vi "ManualMotorControl.vi"() -> ()   [LabVIEW 2021]
uses:
  Controls/Status Lights.ctl
  <vilib>/event_ctls.llb/eventsource.ctl
  <vilib>/event_ctls.llb/lveventtype.ctl
  <vilib>/event_ctls.llb/eventvkey.ctl
  Controls/ManualConttrolCluster.ctl
  Controls/State Machine Data.ctl
  Controls/DAQ Refnums.ctl
  <vilib>/Utility/error.llb/Error Cluster From Error Code.vi
  <vilib>/ErrorRing/Error Ring.xnode
panel:
  in  "Manual Control Cluster":T1 {"Speed" scale=0.0..5.0}
  out "Extend":bool
  out "Stop Button":bool
  out "Retract":bool
  out "Char":i16
  out "VKey":T2
  out "Type":T3=enum."Value Change"
  out "Source":T4 items=["LabVIEW UI"=0, "ActiveX"=1, "User Event"=25]
  out "Mods":cluster{"Num Pad":bool, "Menu Key":bool}
  out "PlatMods":T5
  out "Time":u32
  out "ScanCode":i16
  in  "Simulated Pressure":dbl
  out "Speed":dbl
  out "Actuator Status":T6
  out "Pressure MPa":dbl
  in  "Target Pressure MPa":dbl
  out "Control State":string
  in  "Simulate":bool
  in  "Exit Button":bool
  out "error out":errorcluster
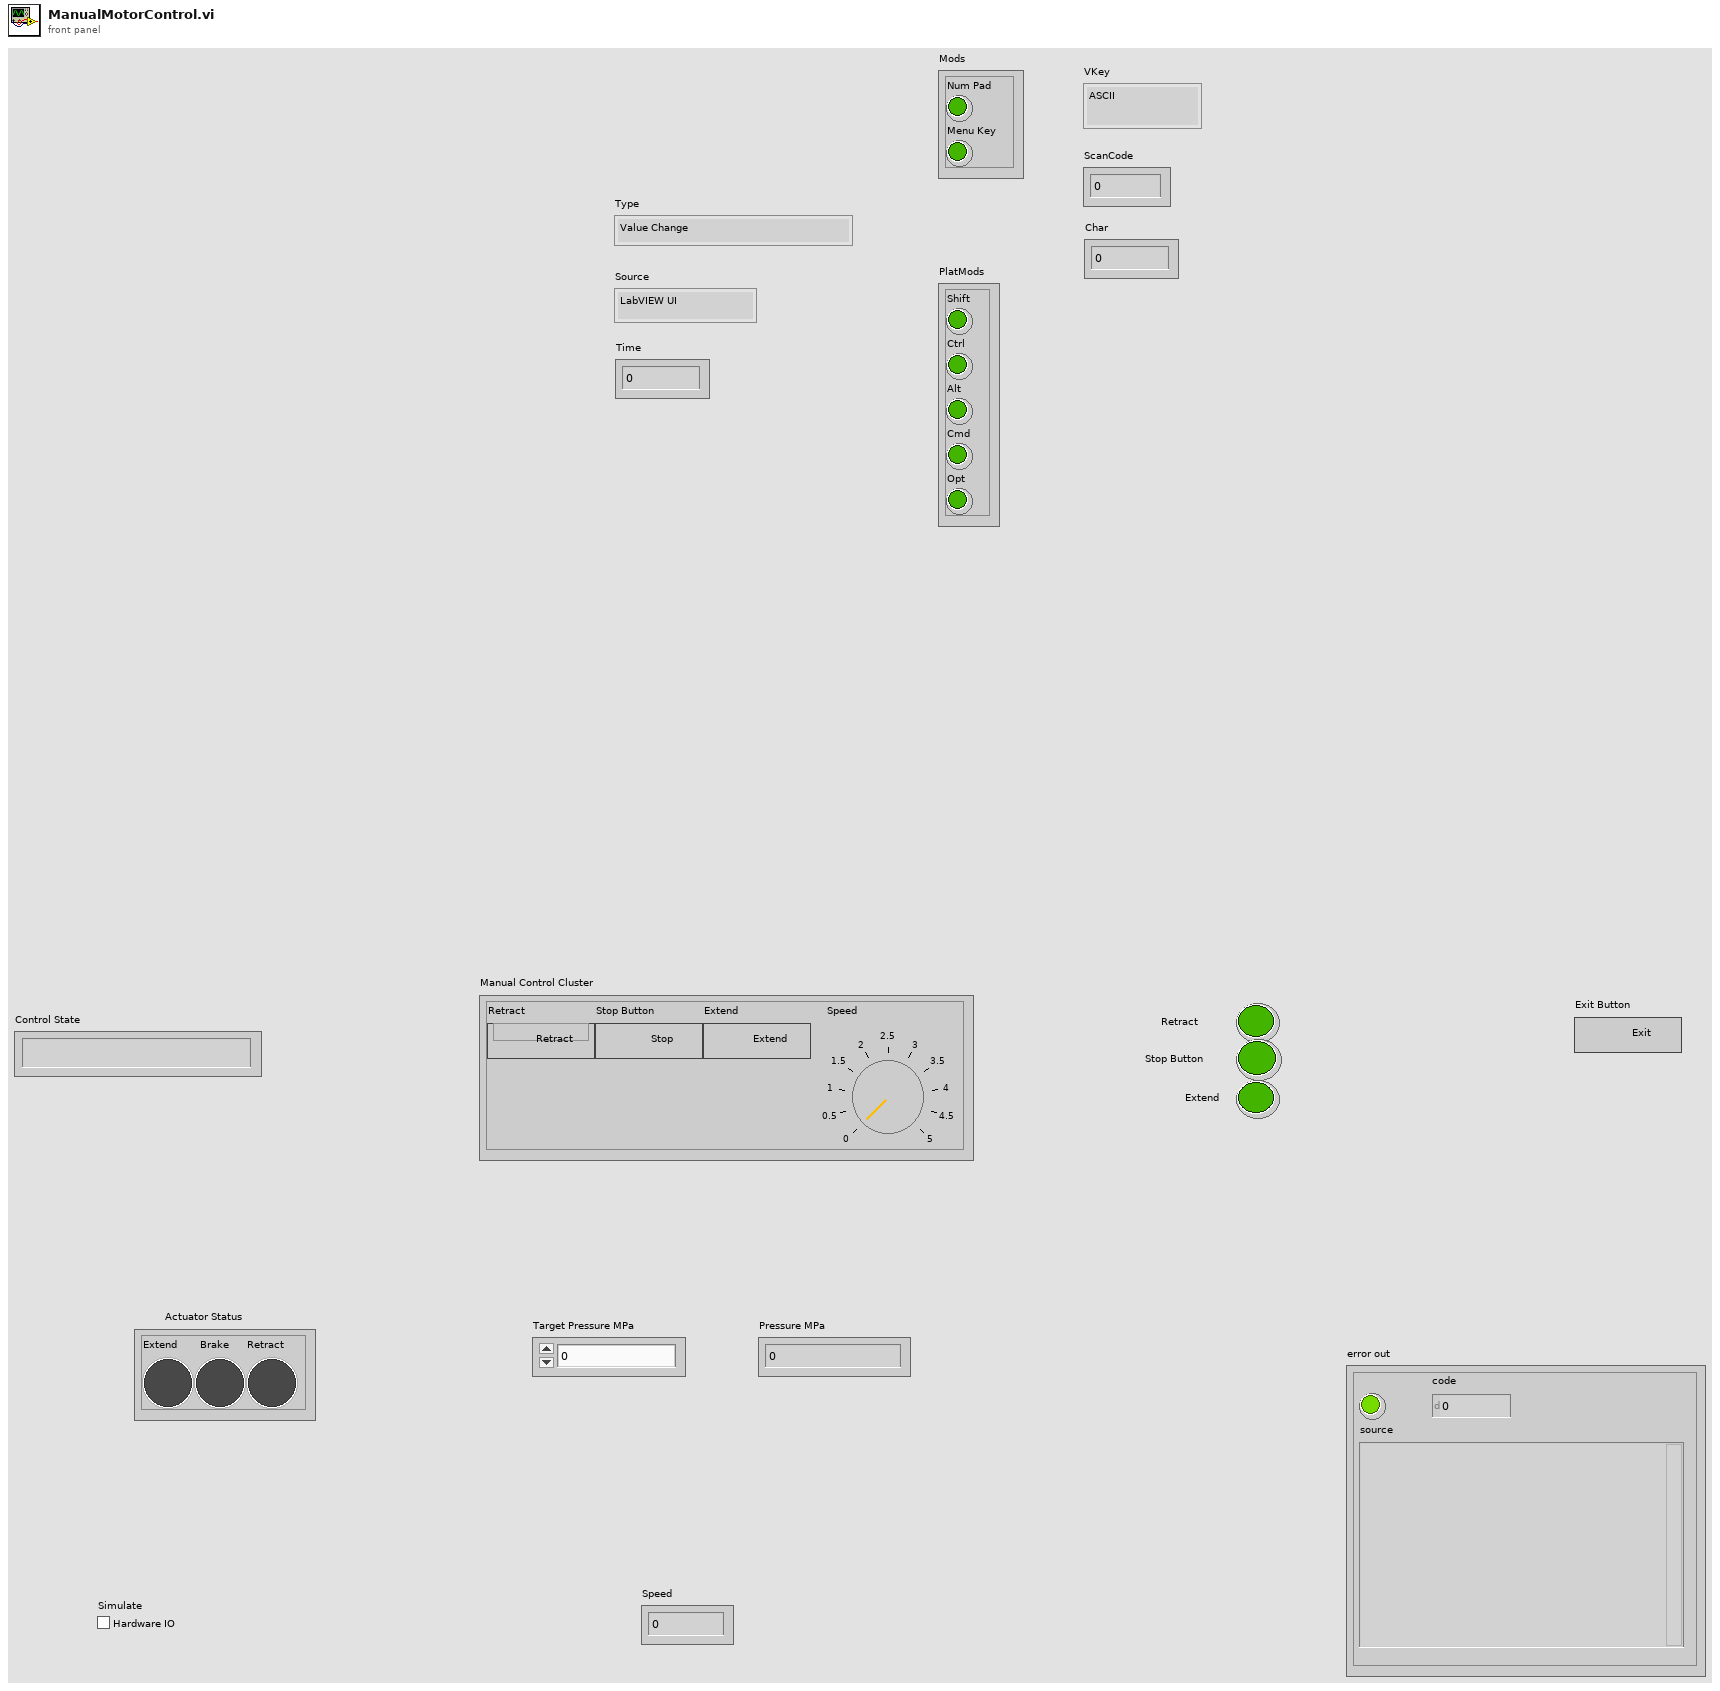
[diagram p1: front panel]
types:
  T1 = typedef "ManualConttrolCluster.ctl" = cluster{"Retract":bool, "Stop Button":bool, "Extend":bool, "Speed":dbl}
  T2 = typedef "eventvkey.ctl" = enum16{"ASCII", "Enter", "Return", "Shift", "Ctrl", "Alt", "Cmd", "Opt", "Caps", "NumLock", "Clear", "Break", "Up", "Down", "Left", "Right", "Insert", "Delete", "Home", "End", "PageUp", "PageDown", "Escape", "Help", "Pause", "ScrollLock", "F1", "F2", "F3", "F4", "F5", "F6", "F7", "F8", "F9", "F10", "F11", "F12", "F13", "F14", "F15", "F16", "F17", "F18", "F19", "F20", "F21", "F22", "F23", "F24", "Play", "VolumeUp", "VolumeDown", "Mute", "Two Byte Char"}
  T3 = typedef "lveventtype.ctl" = enum32{"Null", "Timeout", "Annotation Menu Selection", "Annotation Menu Selection?", "App Instance Close", "App Instance Close?", "Autoscale Range Change", "Bookmark Info Change", "Cell Edit", "Cell Edit?", "Cursor Grab", "Cursor Grab?", "Cursor Menu Selection", "Cursor Menu Selection?", "Cursor Move", "Cursor Release", "Data Change", "Direction Change", "Display State Change", "Drag Ended", "Drag Enter", "Drag Leave", "Drag Over", "Drag Source Update", "Drag Starting", "Drag Starting?", "Drop", "Exec State Change", "Key Down", "Key Down?", "Key Repeat", "Key Repeat?", "Key Up", "Listbox Double Click", "Menu Activation?", "Menu Selection (App)", "Menu Selection? (App)", "Menu Selection (User)", "Mouse Down", "Mouse Down?", "Mouse Enter", "Mouse Leave", "Mouse Move", "Mouse Up", "Mouse Wheel", "NI Security User Change (App)", "Pane Size", "Panel Close", "Panel Close?", "Panel Resize", "Plot Attribute Change", "Scale Range Change", "Shortcut Menu Activation?", "Shortcut Menu Selection (App)", "Shortcut Menu Selection? (App)", "Shortcut Menu Selection (User)", "Tree Double Click", "Tree Drag", "Tree Drag?", "Tree Drop", "Tree Drop?", "Tree Item Close", "Tree Item Close?", "Tree Item Open", "Tree Item Open?", "User Event", "Value Change"}
  T4 = typedef "eventsource.ctl" = u32
  T5 = cluster{"Shift":bool, "Ctrl":bool, "Alt":bool, "Cmd":bool, "Opt":bool}
  T6 = typedef "Status Lights.ctl" = cluster{"Extend":bool, "Brake":bool, "Retract":bool}
  T7 = cluster{"Start Button":refnum<vi>, "Pause Button":refnum<vi>, "Stop Button":refnum<vi>}
  T8 = typedef "State Machine Data.ctl" = cluster{"Control State":string, "Status Message":string, "Speed":dbl, "Pressure":dbl, "Target Pressure":dbl, "Apply Brake Ref":refnum<vi>, "Release Brake Ref":refnum<vi>, "Extend Ref":refnum<vi>, "Retract Ref":refnum<vi>, "Pressure Ref":refnum<vi>, "Data Display Ref":refnum<vi>, "Exit Button Ref":refnum<vi>, "Bool":bool, "Status":T6}
  T9 = typedef "DAQ Refnums.ctl" = cluster{"Direction Ref":refnum<k21>, "Brake Ref":refnum<k21>, "Speed Ref":refnum<k21>, "Pressure Ref":refnum<k21>}
  T10 = typedef "UI Data.ctl" = cluster{"Sampling State":string, "Status Message":string, "Speed":dbl, "Pressure":dbl, "Target Pressure":dbl, "Apply Brake Ref":refnum<vi>, "Release Brake Ref":refnum<vi>, "Extend Ref":refnum<vi>, "Retract Ref":refnum<vi>, "Pressure Ref":refnum<vi>, "Data Display Ref":refnum<vi>, "Exit Button Ref":refnum<vi>, "Speed Pressure Select":bool, "Status":T6}
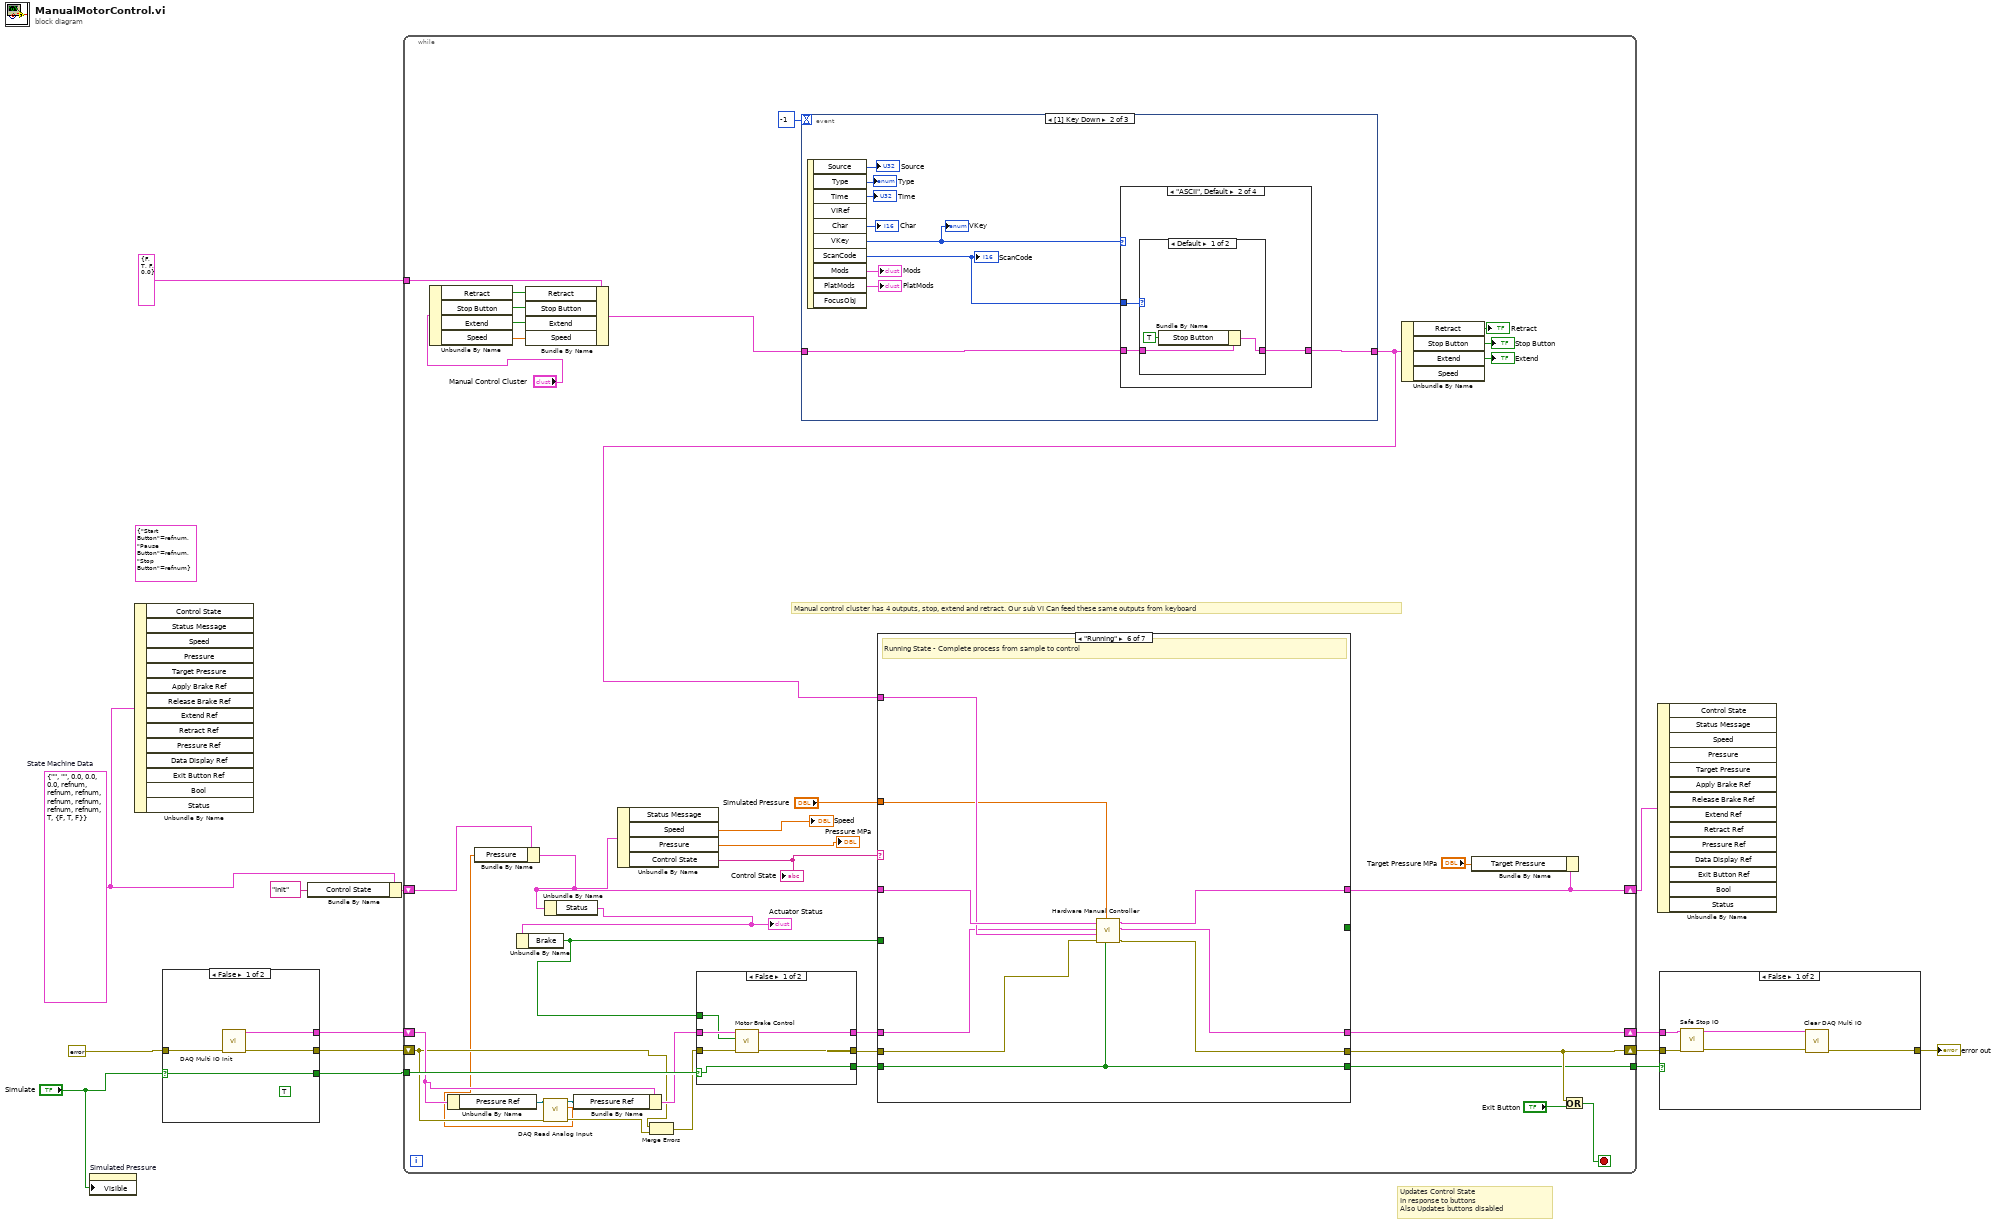
[diagram p0: block diagram]
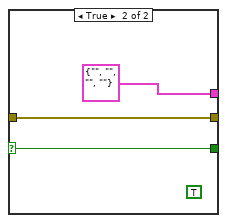
[diagram p3: hidden frame]
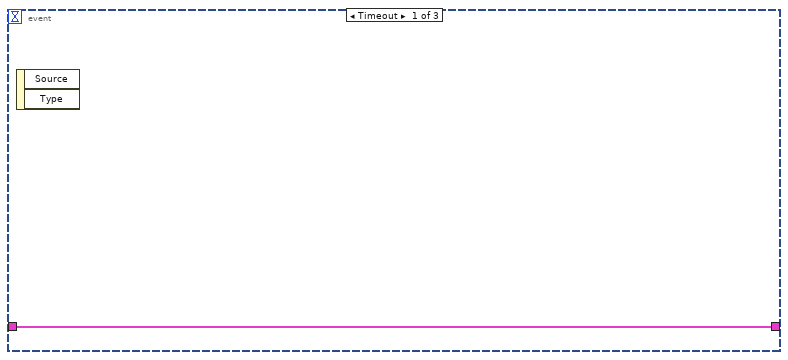
[diagram p4: hidden frame]
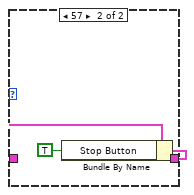
[diagram p6: hidden frame]
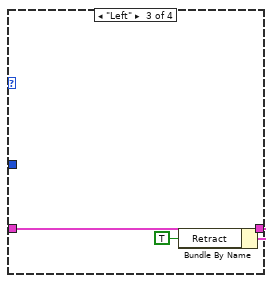
[diagram p7: hidden frame]
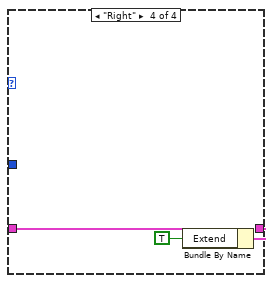
[diagram p8: hidden frame]
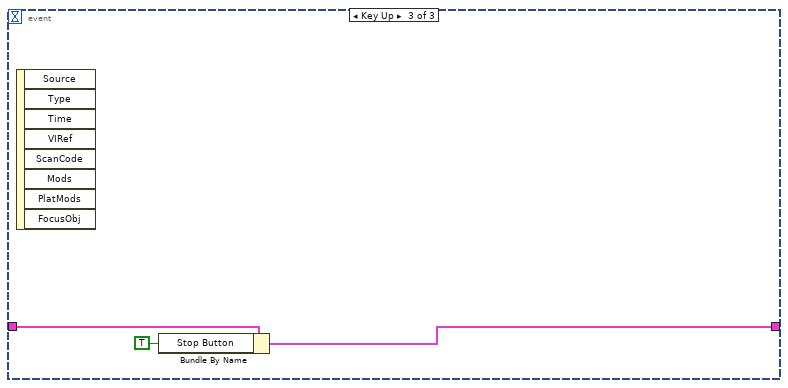
[diagram p9: hidden frame]
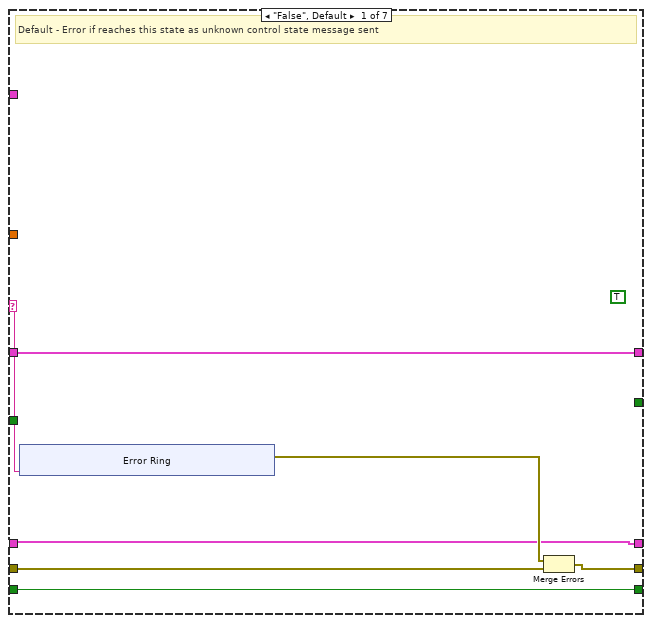
[diagram p11: hidden frame]
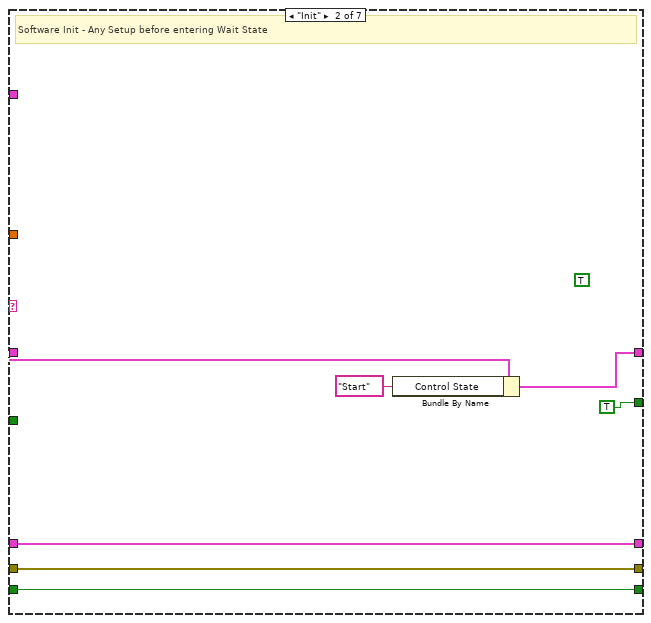
[diagram p12: hidden frame]
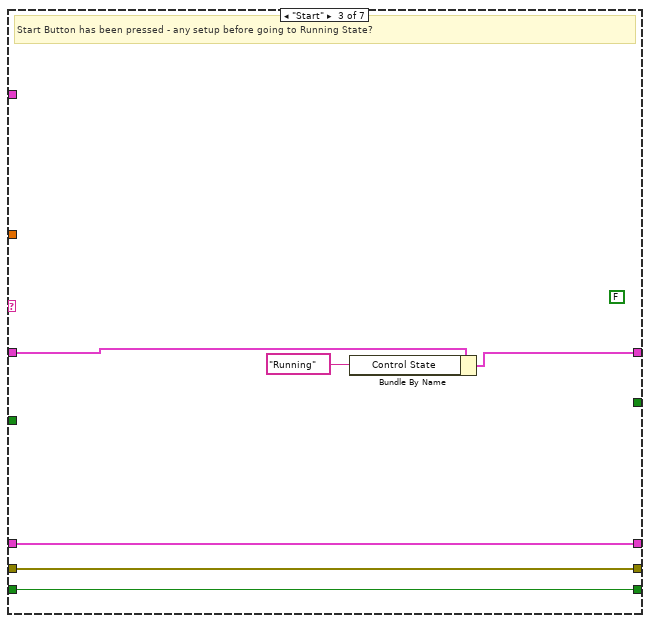
[diagram p13: hidden frame]
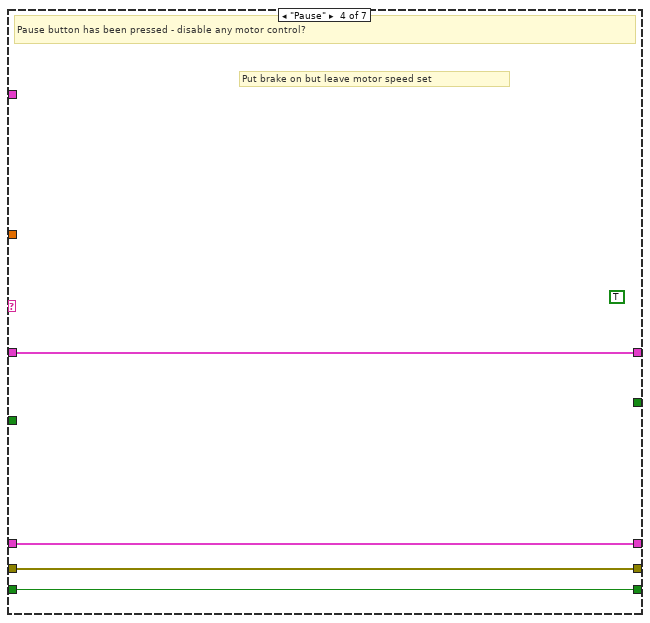
[diagram p14: hidden frame]
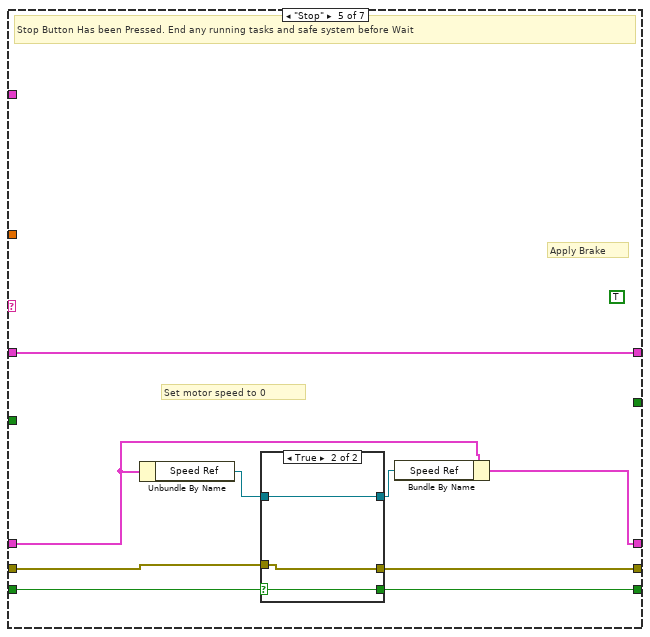
[diagram p15: hidden frame]
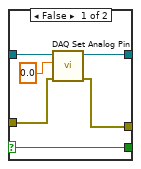
[diagram p16: hidden frame]
diagram:
  (unwired) T7 {"Start Button"=refnum, "Pause Button"=refnum, "Stop Button"=refnum}
  w14 = T8 {"Control State"="", "Status Message"="", "Speed"=0.0, "Pressure"=0.0, "Target Pressure"=0.0, "Apply Brake Ref"=refnum, "Release Brake Ref"=refnum, "Extend Ref"=refnum, "Retract Ref"=refnum, "Pressure Ref"=refnum, "Data Display Ref"=refnum, "Exit Button Ref"=refnum, "Bool"=TRUE, "Status"={"Extend"=FALSE, "Brake"=TRUE, "Retract"=FALSE}}  # State Machine Data
  # "Updates Control State\nIn response to buttons\nAlso Updates buttons disabled"
  n1 = property on="Simulated Pressure" class="DigNum (strict)"("Visible"="Simulate") -> ()  [unwired: 2 in, 2 out]
  n2 = Unbundle By Name(w14) -> ()  [unwired: 14 out]
  n3 = case shown="False" "Simulate" {
    selector: "Simulate" -> [w15 w19]
    tunnel: errorcluster {"status"=FALSE, "code"=0, "source"=""} ("error in") -> [w18 w20]
    tunnel: [w17 w20] -> w10
    tunnel: [w16 T9 {"Direction Ref"="", "Brake Ref"="", "Speed Ref"="", "Pressure Ref"=""} ("DAQ Ref Cluster")] -> w9
    tunnel: [w15 w19] -> w5
    frame False {
      (unwired) TRUE ("Visible")
      n4 = call "DAQ Multi IO Init.vi"("error in"=w18) -> ("error out"=w17:errorcluster, "DAQ Ref Cluster"=w16:T9)  [unwired: 9 in]
    }
    frame True {
      (unwired) TRUE ("Visible")
    }
  }
  n5 = Bundle By Name(cluster=w14, "Control State"="Init") -> (w13:T8)
  n6 = while {
    shift-right: [w39] -> w2
    shift-left: w13 -> [w24]
    shift-right: [w57] -> w6
    shift-left: w10 -> [w27]
    shift-right: [w59] -> w7
    shift-left: w9 -> [w29]
    tunnel: w5 -> [w49]
    tunnel: [w47] -> w4
    tunnel: T1 {"Retract"=FALSE, "Stop Button"=TRUE, "Extend"=FALSE, "Speed"=0.0} ("Manual Control Cluster") -> [w37]
    stop <- w58 stop-if-true
    # "Manual control cluster has 4 outputs, stop, extend and retract. Our sub VI Can feed these same outputs from keyboard"
    n7 = Unbundle By Name("Manual Control Cluster") -> ("Retract"=w35:bool, "Stop Button"=w34:bool, "Extend"=w33:bool, "Speed"=w32:dbl)
    n8 = Unbundle By Name(w29) -> ("Pressure Ref"=w31:refnum<k21>)
    n9 = Bundle By Name(cluster=w37, "Retract"=w35, "Stop Button"=w34, "Extend"=w33, "Speed"=w32) -> (w38:T1)
    n10 = call "DAQ Read Analog Input.vi"("error in"=w27, "task/channels in"=w31) -> ("error out"=w25:errorcluster, "Voltage"=w22:dbl, "task out"=w30:refnum<k21>)  [unwired: 7 in]
    n11 = Bundle By Name(cluster=w24, "Pressure"=w22) -> (w23:T8)
    n12 = Unbundle By Name(w23) -> ("Status"=w53:T6)
    "Actuator Status" <- w53
    n13 = Unbundle By Name(w53) -> ("Brake"=w45:bool)
    n14 = Bundle By Name(cluster=w29, "Pressure Ref"=w30) -> (w28:T9)
    n15 = Unbundle By Name(w23) -> ("Speed"=→"Speed":dbl, "Pressure"=→"Pressure MPa":dbl, "Control State"=w60:string)  [unwired: 1 out]
    "Control State" <- w60
    n16 = Merge Errors(w27, w25) -> (w26:errorcluster)
    n17 = case shown="False" w49 {
      selector: w49 -> [w91 w97]
      tunnel: w26 -> [w96 w98]
      tunnel: [w95 w99] -> w52
      tunnel: [w94 w98] -> w51
      tunnel: w28 -> [w93 w99]
      tunnel: w45 -> [w92 _]
      tunnel: [w91 w97] -> w48
      frame False {
        n18 = call "Motor Brake Control.vi"("error in (no error)"=w96, "Brake"=w92, "DAQ Ref Cluster in"=w93) -> ("error out"=w94:errorcluster, "DAQ Ref Cluster out"=w95:T9)  [unwired: 7 in]
      }
      frame True {
      }
    }
    n19 = event shown="[1] Key Down" {
      selector: _ -> [_ _ _]
      dyn-events: _ -> [_ _ _]
      timeout: -1 -> [_ _ _]
      tunnel: [w61 w63 w89] -> w40
      tunnel: w38 -> [w61 w62 w90]
      event Timeout {
        n20 = event-data() -> ()  [unwired: 1 in, 2 out]
      }
      event Key Down {
        n21 = event-data() -> ("Source"=→"Source":T4, "Type"=→"Type":T3, "Time"=→"Time":u32, "Char"=→"Char":i16, "VKey"=w65:T2, "ScanCode"=w64:i16, "Mods"=→"Mods":cluster{"Num Pad":bool, "Menu Key":bool}, "PlatMods"=→"PlatMods":T5)  [unwired: 1 in, 2 out]
        "VKey" <- w65
        "ScanCode" <- w64
        n22 = case shown="\"ASCII\", Default" w65 {
          tunnel: w64 -> [_ w75 _ _]
          tunnel: [w72 w74 w83 w86] -> w63
          tunnel: w62 -> [w72 w73 w84 w87]
          frame "Enter" {
          }
          frame "ASCII", Default {
            n23 = case shown="Default" w75 {
              tunnel: [w77 w81] -> w74
              tunnel: w73 -> [w78 w80]
              frame Default {
                n24 = Bundle By Name(cluster=w78, "Stop Button"=TRUE) -> (w77:T1)
              }
              frame 57 {
                n25 = Bundle By Name(cluster=w80, "Stop Button"=TRUE) -> (w81:T1)
              }
            }
          }
          frame "Left" {
            n26 = Bundle By Name(cluster=w84, "Retract"=TRUE) -> (w83:T1)
          }
          frame "Right" {
            n27 = Bundle By Name(cluster=w87, "Extend"=TRUE ("Retract")) -> (w86:T1)
          }
        }
      }
      event Key Up {
        n28 = event-data() -> ()  [unwired: 1 in, 8 out]
        n29 = Bundle By Name(cluster=w90, "Stop Button"=TRUE) -> (w89:T1)
      }
    }
    n30 = case shown="\"Running\"" w60 {
      selector: w60 -> [w101 _ _ _ _ _ _]
      tunnel: w23 -> [w103 w116 w123 w128 w139 w157 w159]
      tunnel: [w103 w117 w122 w128 w139 w155 w159] -> w39
      tunnel: [w106 w119 w125 w129 w134 w153 w160] -> w57
      tunnel: w51 -> [w104 w119 w125 w129 w133 w156 w160]
      tunnel: w52 -> [w102 w120 w126 w130 w136 w149 w161]
      tunnel: [w102 w120 w126 w130 w135 w154 w161] -> w59
      tunnel: [_ TRUE ("Reset") _ _ _ _ _] -> _
      tunnel: w45 -> [_ _ _ _ _ _ _]
      tunnel: w48 -> [w100 w114 w121 w127 w132 w150 w158]
      tunnel: [w100 w114 w121 w127 w131 w150 w158] -> w47
      tunnel: "Simulated Pressure" -> [_ _ _ _ _ w151 _]
      tunnel: w40 -> [_ _ _ _ _ w152 _]
      frame "False", Default {
        (unwired) TRUE ("Brake")
        # "Default - Error if reaches this state as unknown control state message sent"
        n31 = xnode "Error Ring"("parameter 0"=w101) -> ("error out"=w105:errorcluster)
        n32 = Merge Errors(w105, w104) -> (w106:errorcluster)
      }
      frame "Init" {
        (unwired) TRUE ("Status.Brake")
        # "Software Init - Any Setup before entering Wait State"
        n33 = Bundle By Name(cluster=w116, "Control State"="Start") -> (w117:T8)
      }
      frame "Start" {
        (unwired) FALSE ("Brake")
        # "Start Button has been pressed - any setup before going to Running State?"
        n34 = Bundle By Name(cluster=w123, "Control State"="Running") -> (w122:T8)
      }
      frame "Pause" {
        (unwired) TRUE ("Brake")
        # "Put brake on but leave motor speed set"
        # "Pause button has been pressed - disable any motor control?"
      }
      frame "Stop" {
        (unwired) TRUE ("Brake")
        # "Apply Brake"
        # "Set motor speed to 0"
        # "Stop Button Has been Pressed. End any running tasks and safe system before Wait"
        n35 = Unbundle By Name(w136) -> ("Speed Ref"=w138:refnum<k21>)
        n36 = case shown="True" w132 {
          selector: w132 -> [w140 w146]
          tunnel: w138 -> [w145 w148]
          tunnel: [w144 w148] -> w137
          tunnel: [w143 w147] -> w134
          tunnel: w133 -> [w142 w147]
          tunnel: [w140 w146] -> w131
          frame False {
            n37 = call "DAQ Set Analog Pin.vi"("error in"=w142, "Voltage"=0.0, "task/channels in"=w145) -> ("error out"=w143:errorcluster, "task out"=w144:refnum<k21>)  [unwired: 6 in, 1 out]
          }
          frame True {
          }
        }
        n38 = Bundle By Name(cluster=w136, "Speed Ref"=w137) -> (w135:T9)
      }
      frame "Running" {
        # "Running State - Complete process from sample to control"
        n39 = call "Hardware Manual Controller.vi"("Simulated"=w150, "Simulated Actual Pressure"=w151, "error in (no error)"=w156, "Manual Control Cluster"=w152, "DAQ Ref Cluster in"=w149, "State Machine Data"=w157) -> ("error out"=w153:errorcluster, "DAQ Ref Cluster out"=w154:T9, "Data Cluster out"=w155:T10)  [unwired: 3 in]
      }
      frame "Wait" {
        # "Wait State - Nothing active should be here"
      }
    }
    n40 = Unbundle By Name(w40) -> ("Retract"=→"Retract":bool, "Stop Button"=→"Stop Button":bool, "Extend"=→"Extend":bool)  [unwired: 1 out]
    n41 = Bundle By Name(cluster=w39, "Target Pressure"="Target Pressure MPa") -> ()  [unwired: 1 out]
    n42 = Or(x=w57, y="Exit Button") -> (x .or. y?=w58:bool)
  }
  n43 = Unbundle By Name(w2) -> ()  [unwired: 14 out]
  n44 = case shown="False" w4 {
    tunnel: [w166 w167] -> w8
    tunnel: w7 -> [w165 _]
    tunnel: w6 -> [w164 w167]
    frame False {
      n45 = call "Safe Stop IO.vi"("error in"=w164, "DAQ Ref Cluster"=w165) -> ("error out"=w162:errorcluster, "DAQ Ref Cluster Out"=w163:T9)  [unwired: 8 in]
      n46 = call "Clear DAQ Multi IO.vi"("error in"=w162, "DAQ Ref"=w163) -> ("error out"=w166:errorcluster)  [unwired: 9 in]
    }
    frame True {
    }
  }
  "error out" <- w8
